vi "subscriber.vi"() -> (0 "error out":errorcluster, 3 "to_rio":cluster{"set_speed":dbl, "set_steering":dbl})   [LabVIEW 2016]
uses:
  <userlib>/ROS for LabVIEW Software/ROS/Code/Console/Servers/ServerSubs/TopicDef.ctl
  <userlib>/ROS for LabVIEW Software/ROS/Code/SubVIs/_ROSDirection.ctl
panel:
  in  "stop":bool
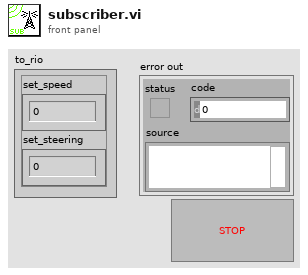
[diagram p1: front panel]
types:
  T1 = typedef "TopicDef.ctl" = cluster{"Topic":string, "Type":string, "Action":T2, "Update (ms)":u16, "queue size":u16}
  T2 = typedef "_ROSDirection.ctl" = enum16{"Node", "Publisher", "Subscriber", "ServiceClient", "ServiceProvider"}
  T3 = typedef "_ROSControl.ctl" = cluster{"topic port":u16, "Node":string, "topic":string, "type":string, "node port":u16, "error ":errorcluster, "Direction":T2, "Update (ms)":u16, "FIFO size":u16}
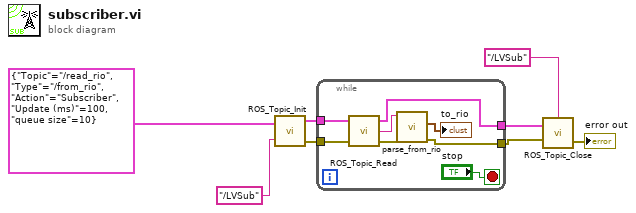
[diagram p0: block diagram]
diagram:
  n1 = call <userlib>:"ROS_Topic_Init.vi"("Definitions"=T1 {"Topic"="/read_rio", "Type"="/from_rio", "Action"=enum."Subscriber", "Update (ms)"=100, "queue size"=10}, "node"="/LVSub") -> ("ROS out"=w7:T3, "error out"=w8:errorcluster)  [unwired: 1 in]
  n2 = while {
    tunnel: w8 -> [w16]
    tunnel: w7 -> [w15]
    tunnel: [w13] -> w6
    tunnel: [w9] -> w1
    stop <- "stop" stop-if-true
    n3 = call <userlib>:"ROS_Topic_Read.vi"("error in (no error)"=w16, "ROS in"=w15) -> ("error out"=w10:errorcluster, "Reply"=w11:string, "ROS out"=w13:T3)  [unwired: 1 in]
    n4 = call "parse_from_rio.vi"("Error In"=w10, "msg in"=w11) -> ("Error Out"=w9:errorcluster, "from_rio"=→"to_rio":cluster{"speed_is":dbl, "steering_is":dbl})  [unwired: 3 in, 1 out]
  }
  n5 = call <userlib>:"ROS_Topic_Close.vi"("error in"=w1, "ROS in"=w6, "node"="/LVSub") -> ("error out"=→"error out":errorcluster)  [unwired: 1 in]
